vi "Simple NLFit.vi"() -> ()   [LabVIEW 2020]
uses:
  <vilib>/Utility/file.llb/Read From Spreadsheet File (DBL).vi
panel:
  out "error out":errorcluster
  out "DataWks":refnum<k7>
  out "Fit":cluster{"data":dbl[], "data":dbl[]}[](graph)
  in  "stop":bool
  out "Input Data":cluster{"data":dbl[], "data":dbl[]}(graph)
  out "Adj. R-Square":dbl
  out "Peak Width":dbl
  out "Peak Center":dbl
  out "SettingsWks":refnum<k7>
  in  "Fitting Function":string(combo)="lorentz"
  in  "Visible":i32(ring) caption="Origin Visible" items=["MAINWND_HIDE"=0, "MAINWND_SHOW"=1, "MAINWND_SHOWMINIMIZED"=2, "MAINWND_SHOWMAXIMIZED"=3, "MAINWND_SHOW_BRING_TO_FRONT"=100]
  out "data filepath":path
  in  "Fitting":bool
  out "ogw path":path
  out "Origin ogw Load":bool
  # "This example shows how to connect to Origin to do curve fitting.\nA simulated data (Lorentzian peak) is sent over to an Origin Analysis Template and the fitting result is then brough back.\nA number of fitting functions can be used to do the fitting and to see the different results. You can see the Lorentzian\nfunction provide the best fit, both visually and from looking at the Adj R-Square values.\n\nRun this vi and choose different Fitting Function and click the Fit button to see the fit results."
  # "Selected Fitting Result Parameters"
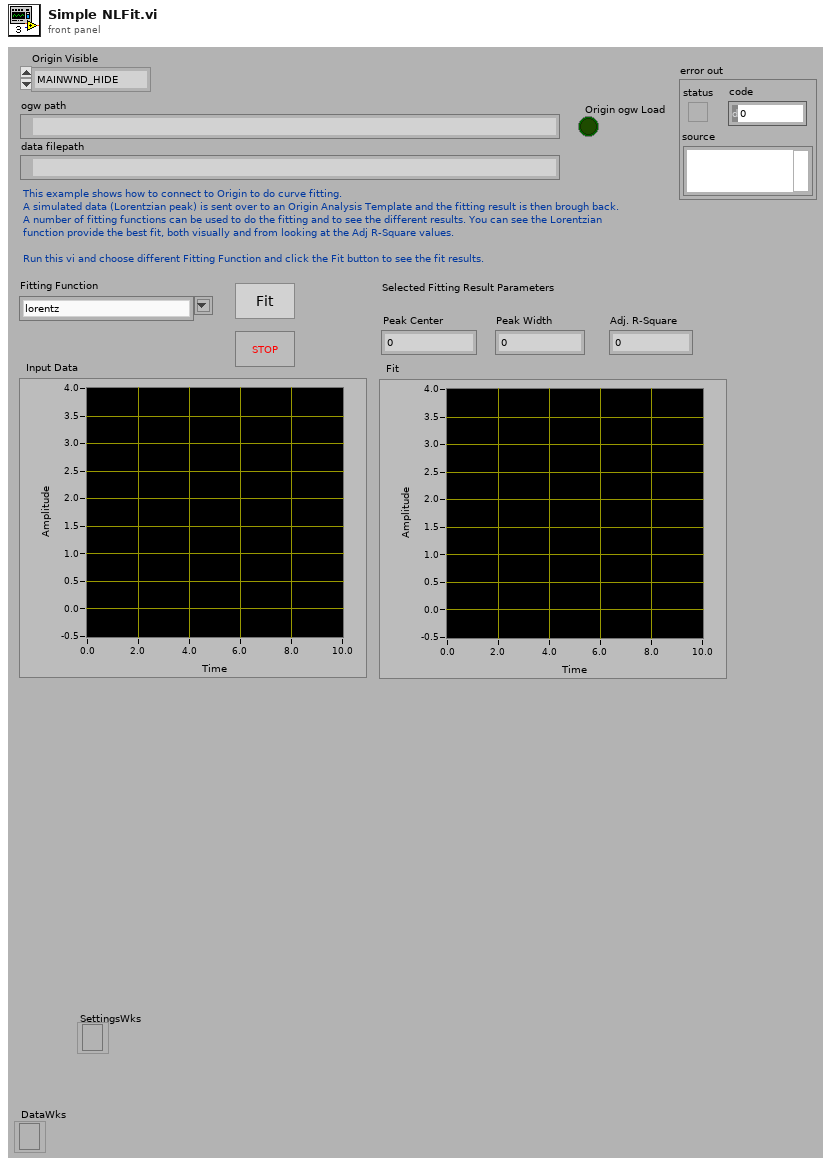
[diagram p1: front panel]
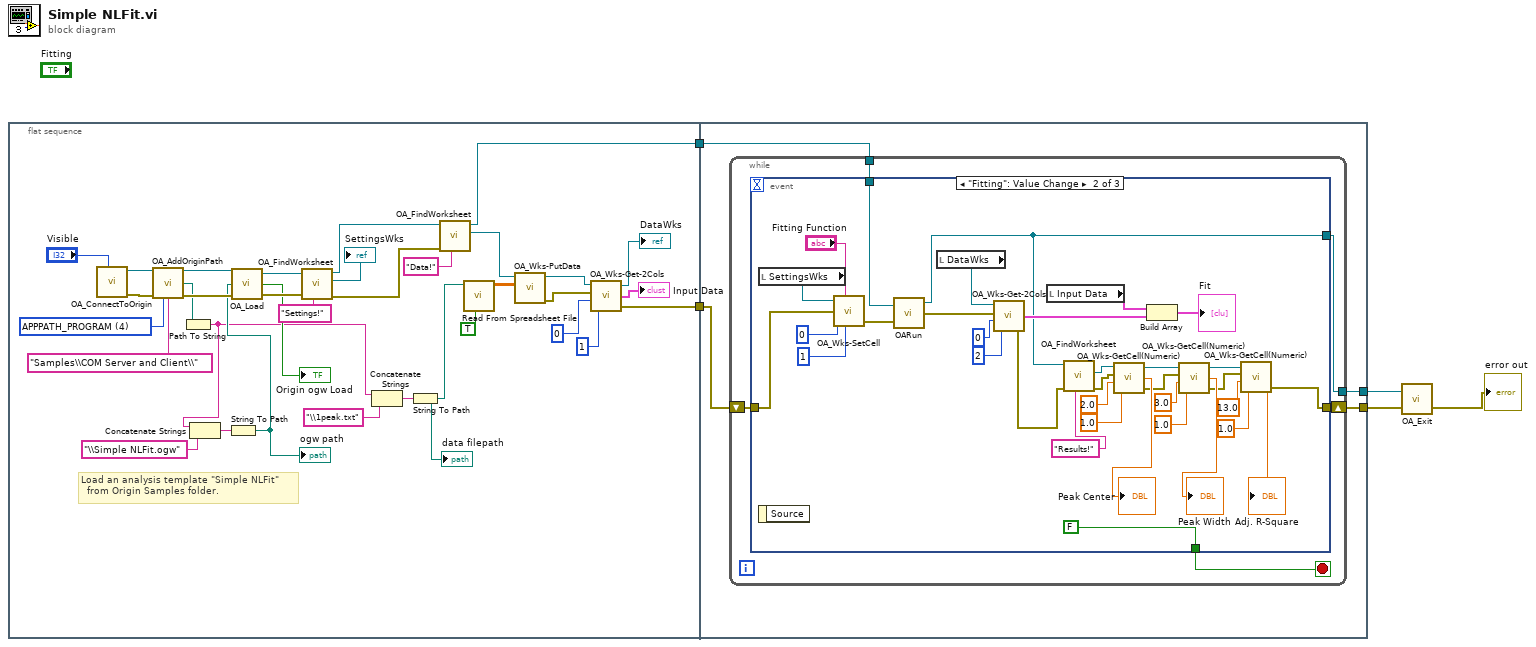
[diagram p0: block diagram]
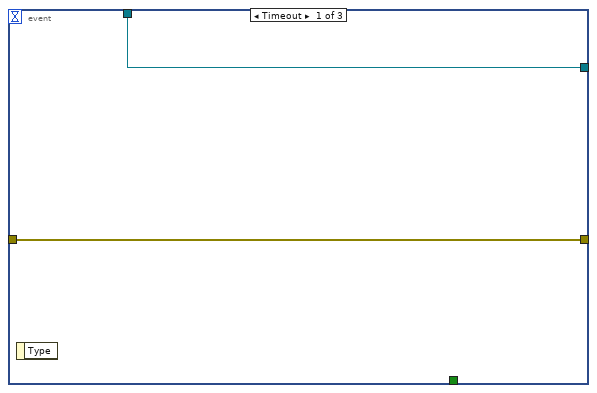
[diagram p2: hidden frame]
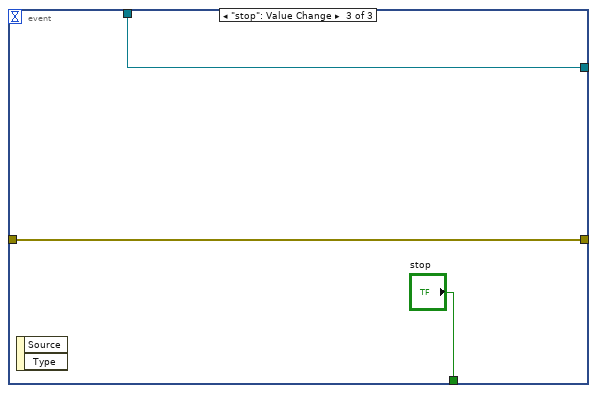
[diagram p3: hidden frame]
diagram:
  n1 = flat-sequence {
    tunnel: [w15] -> w5
    tunnel: [w11] -> w3
    tunnel: w5 -> [w43]
    tunnel: [w42] -> w4
    tunnel: w3 -> [w41]
    tunnel: [w40] -> w2
    frame #0 {
      w37 = 4 items=["APPPATH_USER"=2, "APPPATH_GROUP"=3, "APPPATH_PROGRAM"=4] ("Type")
      # "Load an analysis template \"Simple NLFit\"\n  from Origin Samples folder."
      n2 = call "OA_ConnectToOrigin.vi"("Visible"="Visible") -> ("error out"=w32:errorcluster, "Origin.IOApplication"=w33:refnum<k7>)  [unwired: 7 in]
      n3 = call "OA_AddOriginPath.vi"("Origin.IOApplication"=w33, "error in (no error)"=w32, "Type"=w37, "Filename"="Samples\\COM Server and Client\\") -> ("Origin.IOApplication"=w39:refnum<k7>, "path out"=w27:path, "error out"=w38:errorcluster)  [unwired: 9 in]
      n4 = Path To String(path=w27) -> (string=w23:string)
      n5 = Concatenate Strings(w23, "\\Simple NLFit.ogw" ("string")) -> (w29:string)
      n6 = String To Path(string=w29) -> (path=w28:path)
      "ogw path" <- w28
      n7 = call "OA_Load.vi"("error in (no error)"=w38, "Path"=w28, "Origin.IOApplication"=w39) -> ("error out"=w34:errorcluster, "Load"=→"Origin ogw Load":bool, "Origin.IOApplication"=w35:refnum<k7>)
      n8 = call "OA_FindWorksheet.vi"("Name"="Settings!", "error in (no error)"=w34, "Origin.IOApplication"=w35) -> ("error out"=w16:errorcluster, "Origin.Worksheet"=→"SettingsWks":refnum<k7>, "Origin.IOApplication"=w18:refnum<k7>)  [unwired: 6 in]
      n9 = Concatenate Strings(w23, "\\1peak.txt" ("string")) -> (w25:string)
      n10 = String To Path(string=w25) -> (path=w19:path)
      "data filepath" <- w19
      n11 = call "OA_FindWorksheet.vi"("Name"="Data!", "error in (no error)"=w16, "Origin.IOApplication"=w18) -> ("Origin.Worksheet"=w10:refnum<k7>, "Origin.IOApplication"=w11:refnum<k7>)  [unwired: 6 in, 1 out]
      n12 = call-poly <vilib>:"Read From Spreadsheet File.vi"("transpose (no:F)"=TRUE, "file path (dialog if empty)"=w19) -> ("all rows"=w6:dbl[][])  [unwired: 5 in, 4 out]
      n13 = call "OA_Wks-PutData.vi"("2d Data"=w6, "Origin.Worksheet"=w10) -> ("error out"=w8:errorcluster, "Origin.Worksheet Out"=w9:refnum<k7>)  [unwired: 3 in, 1 out]
      n14 = call "OA_Wks-Get-2Cols.vi"("yCol"=1, "xCol"=0, "error in (no error)"=w8, "Origin.Worksheet"=w9) -> ("error out"=w15:errorcluster, "Bundled Cols"=→"Input Data":cluster{"data":dbl[], "data":dbl[]}, "Origin.Worksheet Dup"=→"DataWks":refnum<k7>)
    }
    frame #1 {
      n15 = while {
        shift-right: [w47] -> w42
        shift-left: w43 -> [w48]
        tunnel: w41 -> [w45]
        tunnel: [w44] -> w40
        stop <- w46 stop-if-true
        n16 = event shown="[1] \"Fitting\": Value Change" {
          selector: _ -> [_ _ _]
          dyn-events: _ -> [_ _ _]
          timeout: _ -> [_ _ _]
          tunnel: w48 -> [w50 w61 w86]
          tunnel: [w50 w51 w86] -> w47
          tunnel: [_ FALSE "stop"] -> w46
          tunnel: w45 -> [w49 w58 w85]
          tunnel: [w49 w52 w85] -> w44
          event Timeout {
            n17 = event-data() -> ()  [unwired: 1 in, 1 out]
          }
          event "Fitting": Value Change {
            n18 = local read "SettingsWks"() -> (w81:refnum<k7>)
            n19 = event-data() -> ()  [unwired: 1 in, 1 out]
            n20 = call "OA_Wks-SetCell.vi"("Origin.Worksheet"=w81, "Data"="Fitting Function", "error in (no error)"=w61, "r1"=0, "c1"=1) -> ("error out"=w54:errorcluster)  [unwired: 2 out]
            n21 = call "OARun.vi"("Origin.IOApplication"=w58, "Error IO"=w54) -> ("Origin.IOApplication"=w52:refnum<k7>, "Error IO Out"=w60:errorcluster)  [unwired: 1 out]
            n22 = local read "DataWks"() -> (w53:refnum<k7>)
            n23 = call "OA_Wks-Get-2Cols.vi"("yCol"=2, "xCol"=0, "error in (no error)"=w60, "Origin.Worksheet"=w53) -> ("error out"=w62:errorcluster, "Bundled Cols"=w57:cluster{"data":dbl[], "data":dbl[]})  [unwired: 1 out]
            n24 = local read "Input Data"() -> (w56:cluster{"data":dbl[], "data":dbl[]})
            n25 = call "OA_FindWorksheet.vi"("Name"="Results!", "error in (no error)"=w62, "Origin.IOApplication"=w52) -> ("error out"=w78:errorcluster, "Origin.Worksheet"=w79:refnum<k7>)  [unwired: 6 in, 1 out]
            n26 = call "OA_Wks-GetCell(Numeric).vi"("c1"=1.0, "r1"=2.0, "error in (no error)"=w78, "Origin.Worksheet"=w79) -> ("error out"=w73:errorcluster, "Data"=→"Peak Center":dbl, "Origin.Worksheet Out"=w74:refnum<k7>)
            n27 = Build Array(w56, w57) -> (→"Fit":cluster{"data":dbl[], "data":dbl[]}[])
            n28 = call "OA_Wks-GetCell(Numeric).vi"("c1"=1.0, "r1"=3.0, "error in (no error)"=w73, "Origin.Worksheet"=w74) -> ("error out"=w68:errorcluster, "Data"=→"Peak Width":dbl, "Origin.Worksheet Out"=w69:refnum<k7>)
            n29 = call "OA_Wks-GetCell(Numeric).vi"("c1"=1.0, "r1"=13.0, "error in (no error)"=w68, "Origin.Worksheet"=w69) -> ("error out"=w51:errorcluster, "Data"=→"Adj. R-Square":dbl)  [unwired: 1 out]
          }
          event "stop": Value Change {
            n30 = event-data() -> ()  [unwired: 1 in, 2 out]
          }
        }
      }
    }
  }
  n31 = call "OA_Exit.vi"("Error IO"=w4, "Origin.IOApplication"=w2) -> ("Error IO Out"=→"error out":errorcluster)  [unwired: 1 out]
